vi "host_with_subvis.vi"() -> ()   [LabVIEW 2014]
uses:
  <vilib>/userdefined/High Color/nirio_resource_hc.ctl
  <instrlib>/niSync/niSync.llb/niSync Initialize (IVI).vi
  <vilib>/FPGAPlugInAG/Dynamic/niLvFpga_Close_Dynamic.vi
  <vilib>/rvi/interface/nirviCloseFPGA/nirviCloseFPGA.xnode
panel:
  in  "AI to plot":i32=3
  in  "trigger  delay":u64
  in  "destination terminal":string(combo)="PXI_Trig1"
  out "Waveform Graph":waveform(dbl)(graph)
  out "Interleaved Raw Data":u64[](array[numeric])
  out "Counts":i16[][](array[numeric])
  out "Voltage":dbl[][](array[numeric])
  in  "num samples":u64=5000
  in  "FPGA name":T1="RIO1" caption="RIO Device"
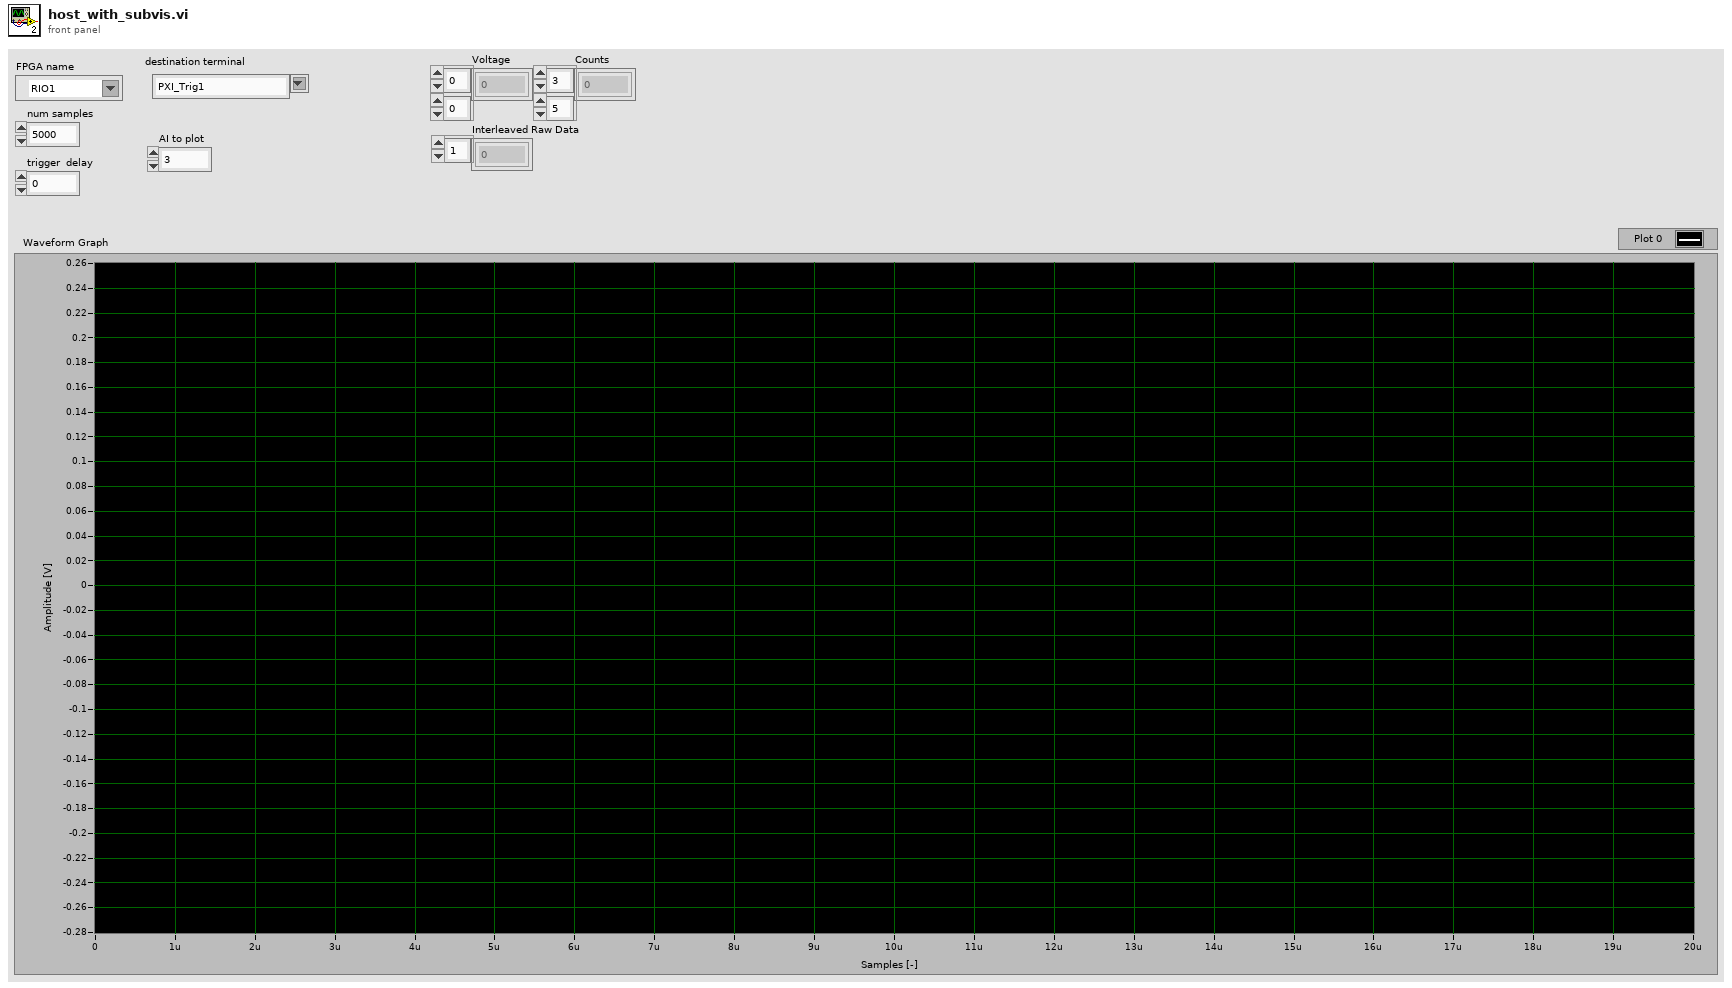
[diagram p1: front panel]
types:
  T1 = typedef "nirio_resource_hc.ctl" = tag
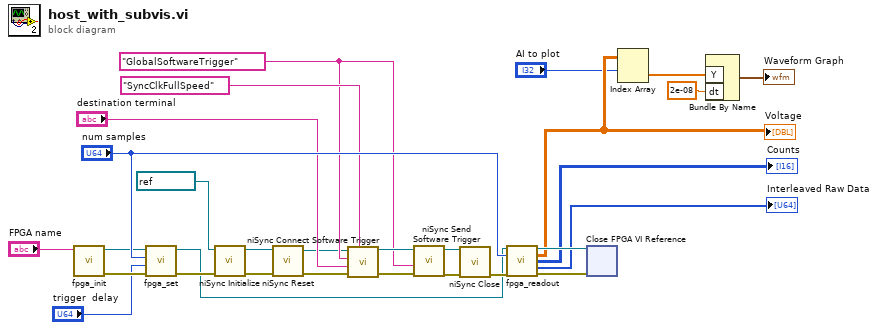
[diagram p0: block diagram]
diagram:
  w16 = "GlobalSoftwareTrigger" ("source terminal")
  n1 = call "fpga_init.vi"("FPGA name"="FPGA name") -> ("error out"=w29:errorcluster, "FPGA VI Reference Out"=w18:refnum<k20>)  [unwired: 9 in]
  n2 = call "fpga_set.vi"("error in"=w29, "trigger  delay"="trigger  delay", "num samples"="num samples", "FPGA VI Reference In"=w18) -> ("error out"=w22:errorcluster, "FPGA VI Reference Out"=w13:refnum<k20>)  [unwired: 6 in]
  n3 = call-poly <instrlib>:"niSync Initialize.vi"("error in (no error)"=w22, "resource name"=refnum<k15> "Sync1") -> ("error out"=w4:errorcluster, "instrument handle out"=w5:refnum<k15>)  [unwired: 8 in]
  n4 = call <instrlib>:"niSync Reset.vi"("error in (no error)"=w4, "instrument handle"=w5) -> ("error out"=w3:errorcluster, "instrument handle out"=w2:refnum<k15>)  [unwired: 8 in]
  n5 = call <instrlib>:"niSync Connect Software Trigger.vi"("synchronization clock"="SyncClkFullSpeed", "error in (no error)"=w3, "destination terminal"="destination terminal", "source terminal"=w16, "instrument handle"=w2) -> ("error out"=w23:errorcluster, "instrument handle out"=w24:refnum<k15>)  [unwired: 5 in]
  n6 = call <instrlib>:"niSync Send Software Trigger.vi"("error in (no error)"=w23, "source terminal"=w16, "instrument handle"=w24) -> ("error out"=w25:errorcluster, "instrument handle out"=w26:refnum<k15>)  [unwired: 7 in]
  n7 = call <instrlib>:"niSync Close.vi"("error in (no error)"=w25, "instrument handle"=w26) -> ("error out"=w21:errorcluster)  [unwired: 9 in]
  n8 = call "fpga_readout.vi"("FPGA VI Reference In"=w13, "samples"="num samples", "error in"=w21) -> ("FPGA Reference Out"=w9:refnum<k20>, "Voltage"=w6:dbl[][], "Counts"=→"Counts":i16[][], "Interleaved Raw Data"=→"Interleaved Raw Data":u64[], "error out"=w14:errorcluster)  [unwired: 8 in]
  "Voltage" <- w6
  n9 = xnode "Close FPGA VI Reference"("FPGA VI Reference In"=w9, "error in"=w14) -> ()  [unwired: 1 out]
  n10 = Index Array(array=w6, index (row)="AI to plot") -> (element=w11:dbl[])  [unwired: 1 in]
  n11 = Bundle By Name("Y"=w11, "dt"=2e-08) -> (→"Waveform Graph":waveform(dbl))  [unwired: 1 in]
